vi "Stop Core.vi"(10 "final error code":i32, 11 "HAL Interface Actor in":refnum<class "HAL Interface Actor.lvclass">) -> (3 "HAL Interface Actor out":refnum<class "HAL Interface Actor.lvclass">)   [LabVIEW 2024, in "HAL Interface Actor.lvlib" / "HAL Interface Actor.lvclass"]
uses:
  HAL Interface Actor.lvclass
  <vilib>/ActorFramework/Time-Delayed Send Message/Time-Delay Override Options.ctl
  HAL Interface Actor.lvclass/HAL Interface Actor.ctl
  <vilib>/ActorFramework/Actor/Actor.lvclass
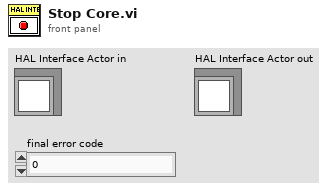
[diagram p1: front panel]
types:
  T1 = typedef "Time-Delay Override Options.ctl" = enum16{"Send next copy now", "Skip next scheduled copy", "Send next copy now and stop all further copies", "Stop all further copies"}
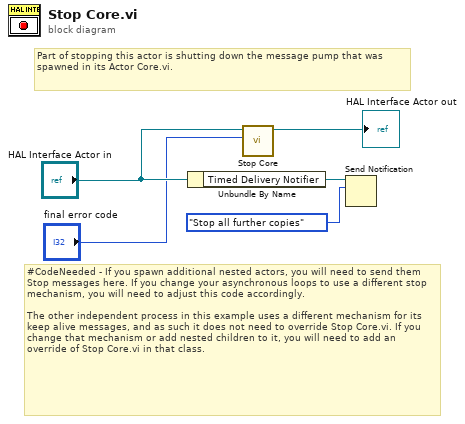
[diagram p0: block diagram]
diagram:
  # "#CodeNeeded - If you spawn additional nested actors, you will need to send them Stop messages here. If you change your asynchronous loops to use a different stop mechanism, you will need to adjust this code accordingly.\n\nThe other independent process in this example uses a different mechanism for its keep alive messages, and as such it does not need to override Stop Core.vi. If you change that mechanism or add nested children to it, you will need to add an override of Stop Core.vi in that class."
  # "Part of stopping this actor is shutting down the message pump that was spawned in its Actor Core.vi."
  n1 = Unbundle By Name("HAL Interface Actor in") -> ("Timed Delivery Notifier"=w3:refnum<notifier>)
  n2 = call-parent "Stop Core.vi"("final error code"="final error code", "Actor in"="HAL Interface Actor in") -> ("Actor out"=→"HAL Interface Actor out":refnum<class "HAL Interface Actor.lvclass">)  [unwired: 9 in]
  n3 = Send Notification(notification=Time-Delay_Override_Options."Stop all further copies", notifier=w3) -> ()  [unwired: 1 in, 2 out]
